vi "Do.vi"(8 "error in (no error)":errorcluster, 10 "Actor in":refnum<class "Actor.lvclass">, 11 "Describe Error Msg":refnum<class "Describe Error Msg.lvclass">) -> (0 "error out":errorcluster, 2 "Actor out":refnum<class "Actor.lvclass">)   [LabVIEW 2014, in "tWorkerCommandRunner.lvlib" / "Describe Error Msg.lvclass"]
doc: "(<B>Filename</B>: Actor Framework.lvlib:Message.lvclass:Do.vi)\n\nDefines what a message does when it is received by an actor. Generally, a message instructs an actor to invoke one of its methods.\n\nBy default, this method does nothing. A child class must override it to define behavior. Create a child class by using the Actor Framework Message Maker dialog box."
uses:
  Describe Error Msg.lvclass
  <vilib>/ActorFramework/Actor/Actor.lvclass
  tWorkerCommandRunner/tWorkerCommandRunner.lvclass
  Describe Error Msg.lvclass/Describe Error Msg.ctl
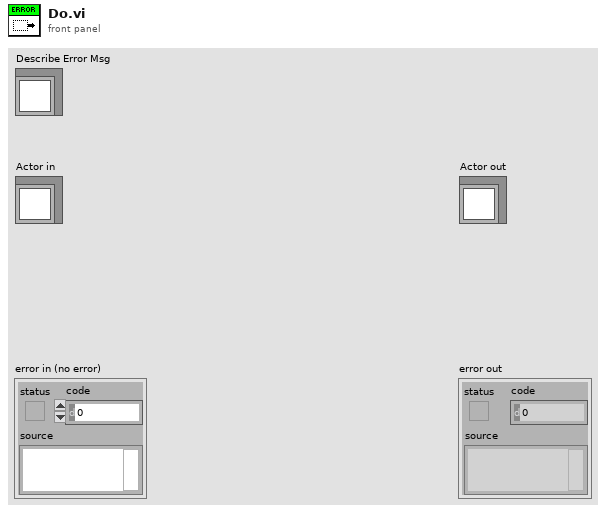
[diagram p1: front panel]
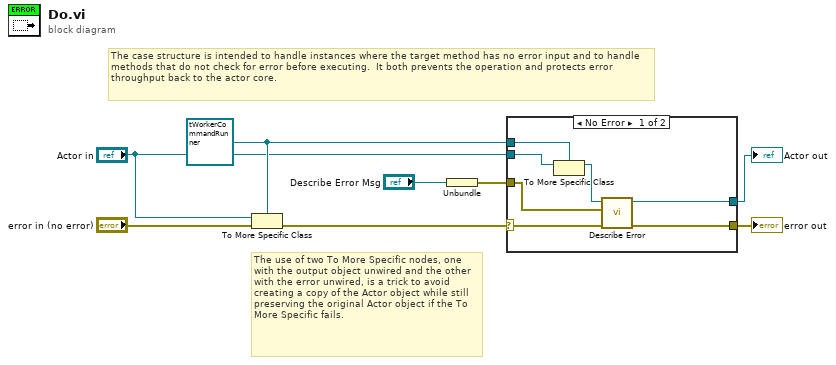
[diagram p0: block diagram]
diagram:
  w7 = refnum<class "tWorkerCommandRunner.lvclass"> refnum ("Actor in")
  # "The use of two To More Specific nodes, one with the output object unwired and the other with the error unwired, is a trick to avoid creating a copy of the Actor object while still preserving the original Actor object if the To More Specific fails."
  # "The case structure is intended to handle instances where the target method has no error input and to handle methods that do not check for error before executing.  It both prevents the operation and protects error throughput back to the actor core."
  n1 = To More Specific Class(target class=w7, reference="Actor in", error in="error in (no error)") -> (error out=w8:errorcluster)  [unwired: 1 out]
  n2 = Unbundle("Describe Error Msg") -> (w3:errorcluster)
  n3 = case shown="No Error" w8 {
    selector: w8 -> [w13 w17]
    tunnel: [w12 w17] -> w1
    tunnel: [w11 w16] -> w2
    tunnel: "Actor in" -> [w15 w16]
    tunnel: w7 -> [w14 _]
    tunnel: w3 -> [w9 _]
    frame No Error {
      n4 = To More Specific Class(target class=w14, reference=w15) -> (specific class reference=w10:refnum<class "tWorkerCommandRunner.lvclass">)  [unwired: 1 in, 1 out]
      n5 = call "Describe Error.vi"("error in (no error)"=w13, "error"=w9, "tWorkerCommandRunner in"=w10) -> ("error out"=w12:errorcluster, "tWorkerCommandRunner out"=w11:refnum<class "tWorkerCommandRunner.lvclass">)  [unwired: 7 in]
    }
    frame Error {
      # "If type check fails, pass the original object out again."
    }
  }
  "error out" <- w1
  "Actor out" <- w2
